vi "Throw Too Many Transfers Error.vi"(7 "source vi name":string, 8 "error in":errorcluster, 10 "num of transfers":i32, 11 "RDMA in":refnum<class "RDMA Transceiver.lvclass">) -> (0 "error out":errorcluster, 3 "RDMA out":refnum<class "RDMA Transceiver.lvclass">)   [LabVIEW 2020, in "RDMA.lvlib" / "RDMA Transceiver.lvclass"]
uses:
  RDMA Transceiver.lvclass
  Errors.ctl
  <vilib>/NI/Memory Manager/Static Errors.lvlib
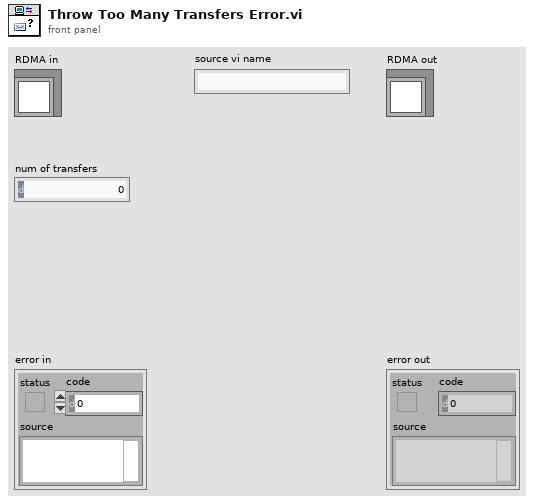
[diagram p1: front panel]
types:
  T1 = typedef "RDMA.lvlib/RDMA Transceiver.lvclass/Errors.ctl" = enum16{"Too Many Transfers", "Size Mismatch", "Unknown Setting"}
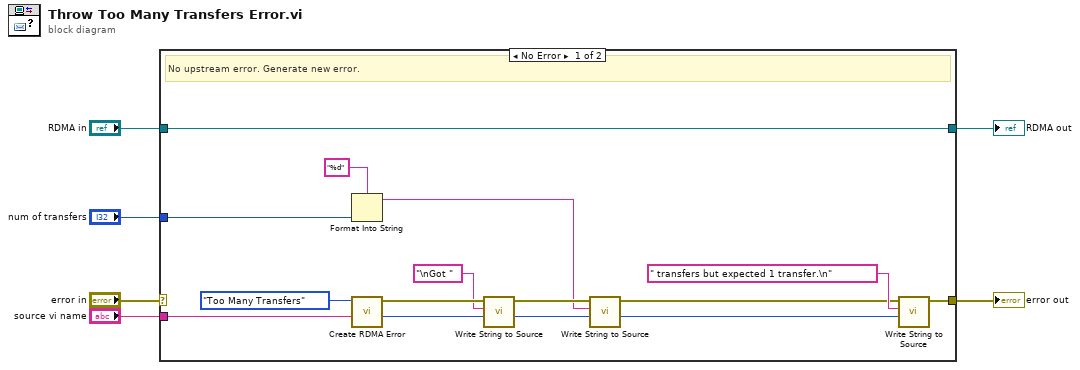
[diagram p0: block diagram]
diagram:
  n1 = case shown="No Error" "error in" {
    selector: "error in" -> [_ w22]
    tunnel: [w16 w22] -> w3
    tunnel: "RDMA in" -> [w21 w23]
    tunnel: [w21 w23] -> w2
    tunnel: "num of transfers" -> [w8 _]
    tunnel: "source vi name" -> [w10 _]
    frame No Error {
      # "No upstream error. Generate new error."
      n2 = Format Into String(format string="%d", w8) -> (resulting string=w9:string)  [unwired: 2 in, 1 out]
      n3 = call "Create RDMA Error.vi"("source vi name"=w10, "error"=Errors."Too Many Transfers" ("Error")) -> ("offset"=w19:i32, "error out"=w18:errorcluster)  [unwired: 8 in]
      n4 = call <vilib>:"Write String to Source.vi"("offset"=w19, "string"="\nGot ", "error in"=w18) -> ("new offset"=w13:i32, "error out"=w14:errorcluster)  [unwired: 7 in]
      n5 = call <vilib>:"Write String to Source.vi"("offset"=w13, "string"=w9, "error in"=w14) -> ("new offset"=w11:i32, "error out"=w12:errorcluster)  [unwired: 7 in]
      n6 = call <vilib>:"Write String to Source.vi"("offset"=w11, "string"=" transfers but expected 1 transfer.\n", "error in"=w12) -> ("error out"=w16:errorcluster)  [unwired: 7 in, 1 out]
    }
    frame Error {
      # "Upstream error. Pass through."
    }
  }
  "error out" <- w3
  "RDMA out" <- w2
